vi "copy.vi"(8 "error in (no error)":errorcluster, 10 "ScriptEventForCopy":refnum<class "ScriptEvent.lvclass">, 11 "PlayFile in":refnum<class "PlayFile.lvclass">) -> (0 "error out":errorcluster, 3 "PlayFile Copy":refnum<class "PlayFile.lvclass">)   [LabVIEW 2011, in "Tools.lvlib" / "Scripting.lvlib" / "PlayFile.lvclass"]
uses:
  PlayFile.lvclass
  ScriptEvent.lvclass
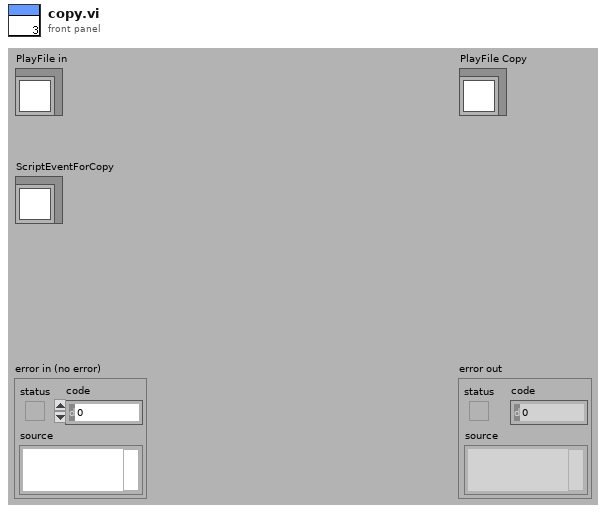
[diagram p1: front panel]
types:
  T1 = enum16{"changeValue", "pulse", "clock", "rampUp", "rampDown", "singleTone", "singleToneRamp", "playFile", "rf", "rfRamp", "delay"}
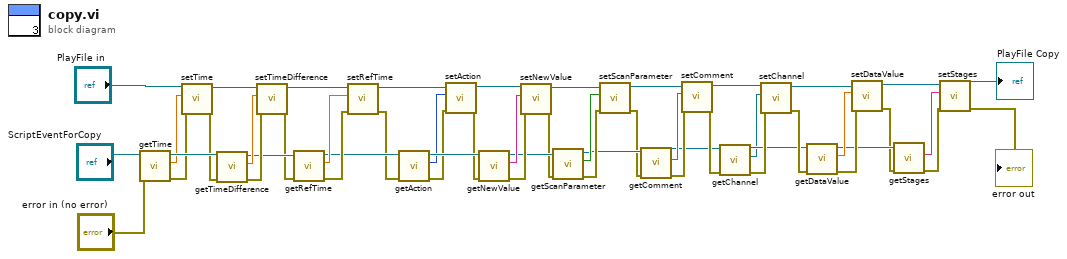
[diagram p0: block diagram]
diagram:
  n1 = call "getTime.vi"("error in (no error)"="error in (no error)", "ScriptEvent.lvclass in"="ScriptEventForCopy") -> ("error out"=w51:errorcluster, "time"=w50:dbl, "ScriptEvent.lvclass out"=w52:refnum<class "ScriptEvent.lvclass">)  [unwired: 7 in]
  n2 = call "setTime.vi"("error in (no error)"=w51, "time"=w50, "ScriptEvent.lvclass in"="PlayFile in") -> ("error out"=w49:errorcluster, "ScriptEvent.lvclass out"=w21:refnum<class "PlayFile.lvclass">)  [unwired: 7 in]
  n3 = call "getTimeDifference.vi"("error in (no error)"=w49, "ScriptEvent.lvclass in"=w52) -> ("error out"=w48:errorcluster, "time difference"=w22:dbl, "ScriptEvent.lvclass out"=w11:refnum<class "ScriptEvent.lvclass">)  [unwired: 7 in]
  n4 = call "setTimeDifference.vi"("error in (no error)"=w48, "time difference"=w22, "ScriptEvent.lvclass in"=w21) -> ("error out"=w10:errorcluster, "ScriptEvent.lvclass out"=w12:refnum<class "PlayFile.lvclass">)  [unwired: 7 in]
  n5 = call "getRefTime.vi"("error in (no error)"=w10, "ScriptEvent.lvclass in"=w11) -> ("error out"=w8:errorcluster, "refTime"=w9:dbl, "ScriptEvent.lvclass out"=w7:refnum<class "ScriptEvent.lvclass">)  [unwired: 7 in]
  n6 = call "setRefTime.vi"("error in (no error)"=w8, "refTime"=w9, "ScriptEvent.lvclass in"=w12) -> ("error out"=w6:errorcluster, "ScriptEvent.lvclass out"=w13:refnum<class "PlayFile.lvclass">)  [unwired: 7 in]
  n7 = call "getAction.vi"("error in (no error)"=w6, "ScriptEvent.lvclass in"=w7) -> ("error out"=w46:errorcluster, "action"=w45:T1, "ScriptEvent.lvclass out"=w47:refnum<class "ScriptEvent.lvclass">)  [unwired: 7 in]
  n8 = call "setAction.vi"("error in (no error)"=w46, "action"=w45, "ScriptEvent.lvclass in"=w13) -> ("error out"=w44:errorcluster, "ScriptEvent.lvclass out"=w20:refnum<class "PlayFile.lvclass">)  [unwired: 7 in]
  n9 = call "getNewValue.vi"("error in (no error)"=w44, "ScriptEvent.lvclass in"=w47) -> ("error out"=w43:errorcluster, "newValue"=w42:string, "ScriptEvent.lvclass out"=w41:refnum<class "ScriptEvent.lvclass">)  [unwired: 7 in]
  n10 = call "setNewValue.vi"("error in (no error)"=w43, "newValue"=w42, "ScriptEvent.lvclass in"=w20) -> ("error out"=w40:errorcluster, "ScriptEvent.lvclass out"=w19:refnum<class "PlayFile.lvclass">)  [unwired: 7 in]
  n11 = call "getScanParameter.vi"("error in (no error)"=w40, "ScriptEvent.lvclass in"=w41) -> ("error out"=w38:errorcluster, "scanParameter"=w39:bool, "ScriptEvent.lvclass out"=w37:refnum<class "ScriptEvent.lvclass">)  [unwired: 7 in]
  n12 = call "setScanParameter.vi"("error in (no error)"=w38, "scanParameter"=w39, "ScriptEvent.lvclass in"=w19) -> ("error out"=w36:errorcluster, "ScriptEvent.lvclass out"=w18:refnum<class "PlayFile.lvclass">)  [unwired: 7 in]
  n13 = call "getComment.vi"("error in (no error)"=w36, "ScriptEvent.lvclass in"=w37) -> ("error out"=w35:errorcluster, "comment"=w34:string, "ScriptEvent.lvclass out"=w32:refnum<class "ScriptEvent.lvclass">)  [unwired: 7 in]
  n14 = call-dynamic "setComment.vi"("error in (no error)"=w35, "comment"=w34, "ScriptEvent.lvclass in"=w18) -> ("error out"=w33:errorcluster, "ScriptEvent.lvclass out"=w17:refnum<class "PlayFile.lvclass">)  [unwired: 7 in]
  n15 = call-dynamic "getChannel.vi"("error in (no error)"=w33, "ScriptEvent.lvclass in"=w32) -> ("error out"=w31:errorcluster, "Channel.lvclass"=w14:refnum<class "Channel.lvclass">, "ScriptEvent.lvclass out"=w29:refnum<class "ScriptEvent.lvclass">)  [unwired: 7 in]
  n16 = call-dynamic "setChannel.vi"("error in (no error)"=w31, "Channel.lvclass"=w14, "ScriptEvent.lvclass in"=w17) -> ("error out"=w30:errorcluster, "ScriptEvent.lvclass out"=w16:refnum<class "PlayFile.lvclass">)  [unwired: 7 in]
  n17 = call "getDataValue.vi"("error in (no error)"=w30, "ScriptEvent.lvclass in"=w29) -> ("error out"=w28:errorcluster, "dataValue"=w27:dbl, "ScriptEvent.lvclass out"=w26:refnum<class "ScriptEvent.lvclass">)  [unwired: 7 in]
  n18 = call "setDataValue.vi"("error in (no error)"=w28, "dataValue"=w27, "ScriptEvent.lvclass in"=w16) -> ("error out"=w25:errorcluster, "ScriptEvent.lvclass out"=w15:refnum<class "PlayFile.lvclass">)  [unwired: 7 in]
  n19 = call "getStages.vi"("error in (no error)"=w25, "ScriptEvent.lvclass in"=w26) -> ("error out"=w24:errorcluster, "Stage"=w23:string)  [unwired: 7 in, 1 out]
  n20 = call-dynamic "setStages.vi"("error in (no error)"=w24, "Stage"=w23, "ScriptEvent.lvclass in"=w15) -> ("error out"=→"error out":errorcluster, "ScriptEvent.lvclass out"=→"PlayFile Copy":refnum<class "PlayFile.lvclass">)  [unwired: 7 in]
